vi "stepper_moveabs.vi"(8 "error in (no error)":errorcluster, 10 "fAbsPos[µm]":sgl min=0 max=4, 11 "reference":refnum<k7>) -> (0 "error out":errorcluster, 3 "reference out":refnum<k7>)   [LabVIEW 2018]
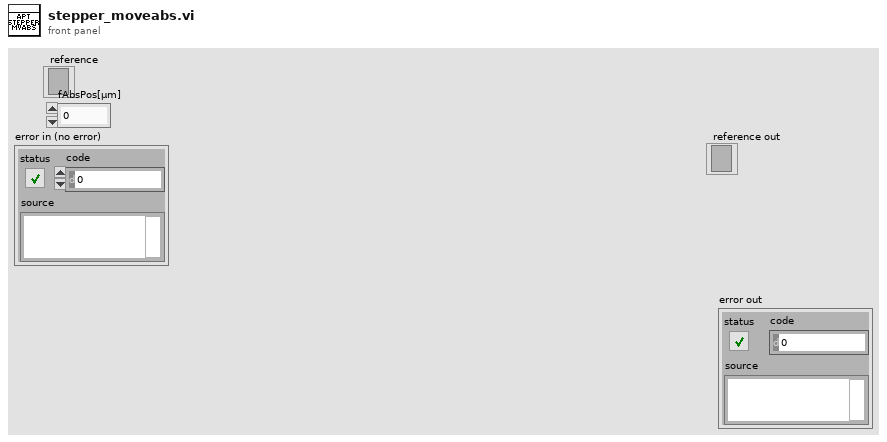
[diagram p1: front panel]
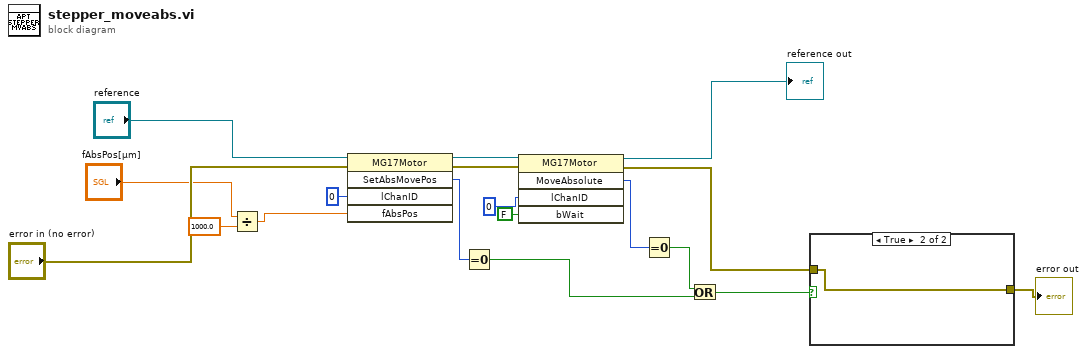
[diagram p0: block diagram]
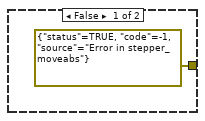
[diagram p2: hidden frame]
diagram:
  n1 = Divide(x="fAbsPos[µm]", y=sgl 1000.0) -> (x/y=w10:sgl)
  n2 = invoke class="MG17Motor" method="SetAbsMovePos"(reference="reference", error in="error in (no error)", "lChanID"=0, "fAbsPos"=w10) -> (reference out=w16:refnum<k7>, error out=w2:errorcluster, "SetAbsMovePos"=w7:i32)  [unwired: 1 in, 2 out]
  n3 = Equal To 0?(x=w7) -> (x = 0?=w5:bool)
  n4 = invoke class="MG17Motor" method="MoveAbsolute"(reference=w16, error in=w2, "lChanID"=0, "bWait"=FALSE) -> (reference out=→"reference out":refnum<k7>, error out=w1:errorcluster, "MoveAbsolute"=w6:i32)  [unwired: 1 in, 2 out]
  n5 = Equal To 0?(x=w6) -> (x = 0?=w4:bool)
  n6 = Or(x=w4, y=w5) -> (x .or. y?=w3:bool)
  n7 = case shown="True" w3 {
    tunnel: [errorcluster {"status"=TRUE, "code"=-1, "source"="Error in stepper_moveabs"} ("error out") w20] -> w8
    tunnel: w1 -> [_ w20]
    frame False {
    }
    frame True {
    }
  }
  "error out" <- w8
